vi "movement back by santimeters.vi"(8 "error in (no error)":errorcluster, 11 "range in santimeters":dbl format="%#_13g") -> (0 "error out":errorcluster)   [LabVIEW 2017]
uses:
  <vilib>/myRIO/Common/Instrument Driver Framework/myRIO v1.0/Encoder/typedefs/Encoder Signal Mode.ctl
  <vilib>/myRIO/Instrument Drivers/Onboard IO/Encoder/typedefs/Encoder Reference.ctl
  <vilib>/myRIO/Common/Instrument Driver Framework/Utilities/typedefs/myRIO Generic Hardware Reference.ctl
  <vilib>/myRIO/Common/Instrument Driver Framework/Utilities/typedefs/Hardware Version Enum.ctl
  <vilib>/myRIO/Common/Instrument Driver Framework/Utilities/typedefs/myRIO v1.0 Reference.ctl
  <vilib>/myRIO/Common/Instrument Driver Framework/Utilities/typedefs/Generic FPGA Reference.ctl
  <vilib>/myRIO/Common/Instrument Driver Framework/myRIO v1.0/Encoder/typedefs/Encoder Channels Enum.ctl
  <vilib>/myRIO/Common/Instrument Driver Framework/myRIO v1.0/Encoder/typedefs/Encoder Configuration v1.0.ctl
  <vilib>/userdefined/High Color/nirio_resource_hc.ctl
  <vilib>/myRIO/Instrument Drivers/Onboard IO/I2C/typedefs/I2C Reference.ctl
  <vilib>/myRIO/Common/Instrument Driver Framework/myRIO v1.0/I2C/typedefs/I2C Channels Enum.ctl
  <vilib>/myRIO/Instrument Drivers/Onboard IO/I2C/typedefs/I2C Configuration.ctl
  <vilib>/myRIO/Instrument Drivers/Onboard IO/I2C/typedefs/I2C Transfer Rate.ctl
  <vilib>/myRIO/Common/Instrument Driver Framework/Utilities/vis/Is FPGA Ref Available.vi
  <vilib>/myRIO/Common/Instrument Driver Framework/myRIO v1.0/Encoder/vis/myRIO v1.1 Open Encoder.vi
  <vilib>/myRIO/Instrument Drivers/Onboard IO/Encoder/vis/Read.vi
  <vilib>/myRIO/Common/Instrument Driver Framework/myRIO v1.0/I2C/vis/myRIO v1.1 Open I2C.vi
  <vilib>/myRIO/Common/Instrument Driver Framework/Utilities/vis/Validate Channels.vi
  <vilib>/myRIO/Common/Instrument Driver Framework/myRIO v1.0/Encoder/vis/myRIO v1.0 Reserve Encoder.vi
  <vilib>/myRIO/Common/Instrument Driver Framework/myRIO v1.0/I2C/vis/myRIO v1.0 Reserve I2C.vi
  <vilib>/myRIO/Common/Instrument Driver Framework/myRIO v1.0/I2C/vis/myRIO v1.0 Close I2C.vi
  <vilib>/myRIO/Common/Instrument Driver Framework/myRIO v1.0/Encoder/vis/myRIO v1.0 Build MUX Configuration Encoder.vi
  <vilib>/myRIO/Common/Instrument Driver Framework/myRIO v1.0/Resource Manager/vis/myRIO v1.0 Reserve Channel List.vi
  <vilib>/myRIO/Common/Instrument Driver Framework/myRIO v1.0/I2C/vis/myRIO v1.0 Build MUX Configuration I2C.vi
  <vilib>/myRIO/Common/Instrument Driver Framework/myRIO v1.0/I2C/vis/myRIO v1.0 Unreserve I2C.vi
  <vilib>/myRIO/Common/Instrument Driver Framework/myRIO v1.0/Resource Manager/vis/myRIO v1.0 Create Configuration List.vi
  <vilib>/myRIO/Common/Instrument Driver Framework/myRIO v1.0/Resource Manager/vis/myRIO v1.0 Reserve Channel.vi
  <vilib>/myRIO/Common/Instrument Driver Framework/myRIO v1.0/Resource Manager/vis/myRIO v1.0 Unreserve Channel.vi
  <vilib>/myRIO/Common/Instrument Driver Framework/myRIO v1.0/Resource Manager/vis/myRIO v1.0 Unreserve Channel List.vi
  <vilib>/myRIO/Common/Instrument Driver Framework/myRIO v1.0/Resource Manager/vis/myRIO v1.0 Build Mutex Name.vi
  <vilib>/Utility/VariantDataType/GetNumericInfo.vi
  <vilib>/Utility/error.llb/Error Cluster From Error Code.vi
  <vilib>/myRIO/Common/Instrument Driver Framework/myRIO v1.0/myRIO v1.1 Open.vi
  <vilib>/myRIO/Common/Instrument Driver Framework/Utilities/vis/IO Manager.vi
  <vilib>/myRIO/Common/Instrument Driver Framework/Utilities/vis/Configuration Manager.vi
  <vilib>/myRIO/Common/Instrument Driver Framework/myRIO v1.0/Resource Manager/vis/myRIO v1.0 Configure IO.vi
  <vilib>/myRIO/Common/Instrument Driver Framework/myRIO v1.0/myRIO v1.0 Close.vi
  <vilib>/myRIO/Common/Instrument Driver Framework/myRIO v1.0/Encoder/vis/myRIO v1.0 Configure Encoder.vi
  <vilib>/myRIO/Common/Instrument Driver Framework/myRIO v1.0/Encoder/vis/myRIO v1.0 Read Encoder.vi
  <vilib>/myRIO/Common/Instrument Driver Framework/myRIO v1.0/DIO/vis/myRIO v1.0 Write DIO.vi
  <vilib>/myRIO/Common/Instrument Driver Framework/myRIO v1.0/I2C/vis/myRIO v1.0 Shutdown I2C.vi
  <vilib>/myRIO/Instrument Drivers/Onboard IO/I2C/vis/myRIO I2C Open.xnode
  <vilib>/myRIO/Express VI/Onboard IO/Encoder/Encoder Express VI.xnode
  <vilib>/myRIO/Instrument Drivers/Onboard IO/Encoder/vis/myRIO Encoder Open.xnode
  <vilib>/myRIO/Instrument Drivers/Onboard IO/I2C/I2C.lvlib
  <vilib>/myRIO/Instrument Drivers/Onboard IO/Encoder/Encoder.lvlib
  <vilib>/myRIO/Instrument Drivers/Onboard IO/DIO/DIO.lvlib
panel:
  out "main angle":ext
  out "axis Z(after)":ext
  out "zero angle":ext
  out "left":dbl
  out "right":dbl
  out "axis Z(paste)":ext
  in  "Stop Button":bool
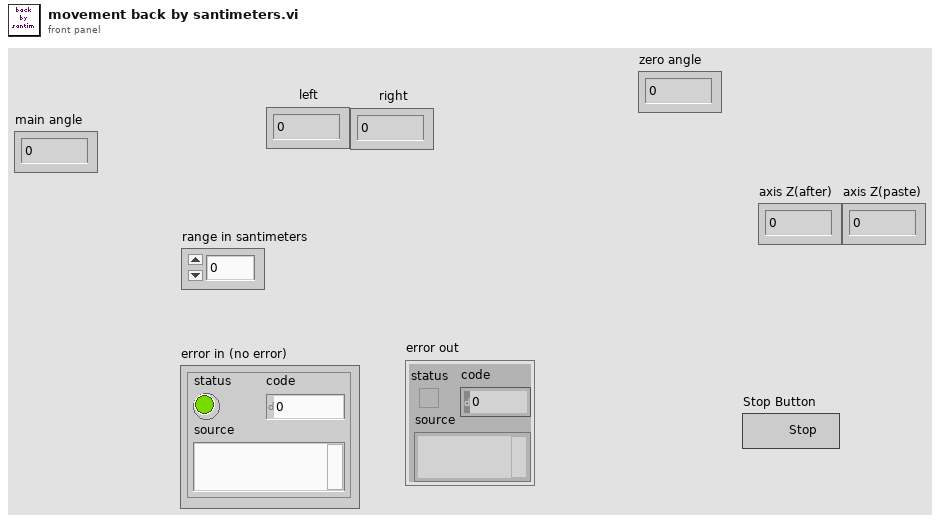
[diagram p1: front panel]
types:
  T1 = typedef "DIO.lvlib/DIO Reference.ctl" = cluster{"myRIO Reference":T2, "DIO Channels List":T6}
  T2 = typedef "myRIO Generic Hardware Reference.ctl" = cluster{"myRIO Model":T3, "myRIO Hardware Reference":T4}
  T3 = typedef "Hardware Version Enum.ctl" = enum16{"Unknown", "myRIO-1900", "myRIO-1950", "roboRIO", "NI ELVIS RIO CM"}
  T4 = typedef "myRIO v1.0 Reference.ctl" = cluster{"Generic FPGA Reference":T5, "Allow multiple opens":bool}
  T5 = typedef "Generic FPGA Reference.ctl" = refnum<k20>
  T6 = typedef "DIO Channels List.ctl" = T7[]
  T7 = typedef "DIO Channels Enum.ctl" = enum16{"Not Connected", "C/DIO0", "C/DIO1", "C/DIO2", "C/DIO3", "C/DIO4", "C/DIO5", "C/DIO6", "C/DIO7", "A/DIO0", "A/DIO1", "A/DIO2", "A/DIO3", "A/DIO4", "A/DIO5", "A/DIO6", "A/DIO7", "A/DIO8", "A/DIO9", "A/DIO10", "A/DIO11", "A/DIO12", "A/DIO13", "A/DIO14", "A/DIO15", "B/DIO0", "B/DIO1", "B/DIO2", "B/DIO3", "B/DIO4", "B/DIO5", "B/DIO6", "B/DIO7", "B/DIO8", "B/DIO9", "B/DIO10", "B/DIO11", "B/DIO12", "B/DIO13", "B/DIO14", "B/DIO15", "LED0", "LED1", "LED2", "LED3", "Button0", "DIO/DIO0", "DIO/DIO1", "DIO/DIO2", "DIO/DIO3", "DIO/DIO4", "DIO/DIO5", "DIO/DIO6", "DIO/DIO7", "DIO/DIO8", "DIO/DIO9", "SPI/CS0", "SPI/CS1", "SPI/CS2", "SPI/CS3", "LED RADIO (Green)", "LED RADIO (Red)", "LED COMM (Green)", "LED COMM (Red)", "LED MODE (Green)", "LED MODE (Red)"}
  T8 = typedef "I2C.lvlib/I2C Reference.ctl" = cluster{"myRIO Reference":T2, "I2C Channels Enum":T9, "I2C Configuration":T10}
  T9 = typedef "I2C Channels Enum.ctl" = enum16{"Not Connected", "A/I2C", "B/I2C", "I2C/I2C"}
  T10 = typedef "I2C.lvlib/I2C Configuration.ctl" = cluster{"I2C Transfer Rate":T11}
  T11 = typedef "I2C.lvlib/I2C Transfer Rate.ctl" = enum16{"Standard mode (100 kbps)", "Fast mode (400 kbps)"}
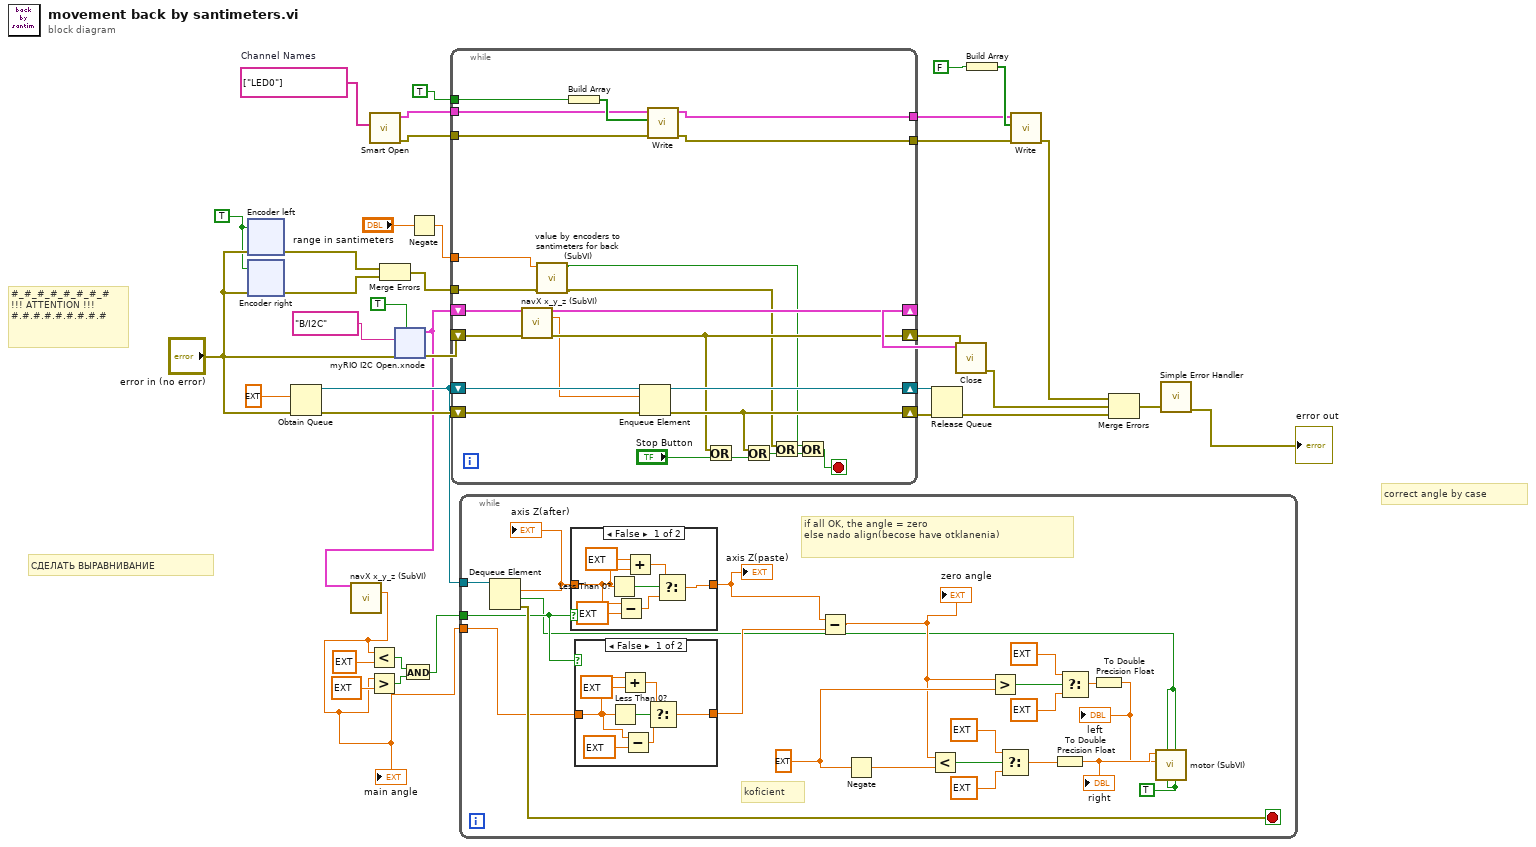
[diagram p0: block diagram]
diagram:
  w9 = tag[] ["LED0"]  # Channel Names
  w10 = TRUE ("Reset Counter")
  # "СДЕЛАТЬ ВЫРАВНИВАНИЕ"
  # "correct angle by case"
  # "#_#_#_#_#_#_#_#\n!!! ATTENTION !!!\n#.#.#.#.#.#.#.#.#"
  n1 = xnode ("Encoder left")("error in (no error)"="error in (no error)", "Reset Counter"=w10) -> ("error out"=w15:errorcluster)  [unwired: 3 out]
  n2 = xnode ("Encoder right")("error in (no error)"="error in (no error)", "Reset Counter"=w10) -> ("error out"=w14:errorcluster)  [unwired: 3 out]
  n3 = Obtain Queue(element data type=ext 0.0 ("value Z"), error in (no error)="error in (no error)") -> (queue out=w25:refnum<queue>, error out=w37:errorcluster)  [unwired: 3 in, 1 out]
  n4 = call <vilib>:"Smart Open.vi"("Channel Names"=w9) -> ("error out"=w4:errorcluster, "DIO Ref Out"=w5:T1)  [unwired: 9 in]
  n5 = Merge Errors(w15, w14) -> (w13:errorcluster)
  n6 = xnode "myRIO I2C Open.xnode"("error in (no error)"="error in (no error)", "Allow multiple opens?"=TRUE, "Channel Name"=tag "B/I2C") -> ("error out"=w30:errorcluster, "I2C Ref Out"=w23:T8)
  n7 = call "navX x_y_z (SubVI).vi"("I2C Ref Out in"=w23) -> ("value Z"=w20:ext)  [unwired: 10 in, 4 out]
  "main angle" <- w20
  n8 = Less?(x=w20, y=ext 90.0) -> (x < y?=w18:bool)
  n9 = Greater?(x=w20, y=ext -90.0) -> (0:w21:bool)
  n10 = And(x=w18, y=w21) -> (x .and. y?=w17:bool)
  n11 = Negate(x="range in santimeters") -> (-x=w11:dbl)
  n12 = while {
    shift-right: [w55] -> w35
    shift-left: w37 -> [w60]
    shift-right: [w59] -> w36
    shift-left: w25 -> [w61]
    shift-right: [w56] -> w31
    shift-left: w23 -> [w57]
    shift-right: [w52] -> w29
    shift-left: w30 -> [w53]
    tunnel: w13 -> [w44]
    tunnel: w11 -> [w47]
    tunnel: TRUE -> [w43]
    tunnel: w5 -> [w41]
    tunnel: w4 -> [w40]
    tunnel: [w39] -> w3
    tunnel: [w38] -> w2
    stop <- w49 stop-if-true
    n13 = call "navX x_y_z (SubVI).vi"("I2C Ref Out in"=w57, "error in (no error)"=w53) -> ("I2C Ref Out out"=w56:T8, "value Z"=w51:ext, "error out"=w52:errorcluster)  [unwired: 9 in, 2 out]
    n14 = call "value by encoders to santimeters for back (SubVI).vi"("error in (no error)"=w44, "range in"=w47) -> ("error out"=w45:errorcluster, "value >= range"=w46:bool)  [unwired: 7 in, 1 out]
    n15 = Build Array(w43) -> (w42:bool[])
    n16 = Enqueue Element(queue=w61, element=w51, error in (no error)=w60) -> (queue out=w59:refnum<queue>, error out=w55:errorcluster)  [unwired: 1 in, 1 out]
    n17 = call <vilib>:"Write.vi"("error in (no error)"=w40, "Values"=w42, "DIO Ref In"=w41) -> ("error out"=w38:errorcluster, "DIO Ref Out"=w39:T1)  [unwired: 6 in]
    n18 = Or(x=w52, y="Stop Button") -> (x .or. y?=w54:bool)
    n19 = Or(x=w55, y=w54) -> (x .or. y?=w50:bool)
    n20 = Or(x=w45, y=w50) -> (x .or. y?=w48:bool)
    n21 = Or(x=w46, y=w48) -> (x .or. y?=w49:bool)
  }
  n22 = while {
    tunnel: w25 -> [w83]
    tunnel: w20 -> [w67]
    tunnel: w17 -> [w66]
    stop <- w82 stop-if-true
    w65 = TRUE ("M1 (Pin 26)")
    w75 = ext 1.0 ("y")
    # "koficient"
    # "if all OK, the angle = zero\nelse nado align(becose have otklanenia)"
    n23 = Dequeue Element(queue=w83) -> (element=w69:ext, timed out?=w64:bool, error out=w82:errorcluster)  [unwired: 2 in, 1 out]
    "axis Z(after)" <- w69
    n24 = case shown="False" w66 {
      tunnel: [w97 w99] -> w70
      tunnel: w69 -> [w93 w99]
      frame False {
        n25 = Less Than 0?(x=w93) -> (x < 0?=w98:bool)
        n26 = Subtract(x=w93, y=ext 180.0) -> (x-y=w94:ext)
        n27 = Add(x=ext 180.0, y=w93) -> (x+y=w96:ext)
        n28 = Select(t=w96, s=w98, f=w94) -> (s? t:f=w97:ext)
      }
      frame True {
      }
    }
    "axis Z(paste)" <- w70
    n29 = case shown="False" w66 {
      tunnel: [w89 w91] -> w68
      tunnel: w67 -> [w86 w91]
      frame False {
        n30 = Less Than 0?(x=w86) -> (x < 0?=w90:bool)
        n31 = Add(x=w86, y=ext 180.0) -> (x+y=w88:ext)
        n32 = Subtract(x=w86, y=ext 180.0) -> (x-y=w87:ext)
        n33 = Select(t=w88, s=w90, f=w87) -> (s? t:f=w89:ext)
      }
      frame True {
      }
    }
    n34 = Subtract(x=w70, y=w68) -> (x-y=w71:ext)
    "zero angle" <- w71
    n35 = Negate(x=w75) -> (-x=w74:ext)
    n36 = Less?(x=w71, y=w74) -> (x < y?=w78:bool)
    n37 = Greater?(x=w71, y=w75) -> (0:w81:bool)
    n38 = Select(t=ext 0.2 ("y"), s=w78, f=ext 0.30000000000000000001 ("y")) -> (s? t:f=w72:ext)
    n39 = To Double Precision Float(number=w72) -> (double precision float=w63:dbl)
    "right" <- w63
    n40 = Select(t=ext 0.2 ("y"), s=w81, f=ext 0.30000000000000000001 ("y")) -> (s? t:f=w73:ext)
    n41 = To Double Precision Float(number=w73) -> (double precision float=w62:dbl)
    "left" <- w62
    n42 = call "motor (SubVI).vi"("M1 (Pin 26)"=w65, "M1 (Pin 25)"=w64, "M0 (Pin 23)"=w65, "M0 (Pin 21)"=w64, "PWM1"=w62, "PWM0"=w63) -> ()  [unwired: 5 in, 1 out]
  }
  n43 = Release Queue(queue=w36, error in (no error)=w35) -> (error out=w26:errorcluster)  [unwired: 1 in, 2 out]
  n44 = call <vilib>:"Close.vi"("error in (no error)"=w29, "I2C Ref In"=w31) -> ("error out"=w27:errorcluster)  [unwired: 9 in]
  n45 = Build Array(FALSE) -> (w8:bool[])
  n46 = call <vilib>:"Write.vi"("error in (no error)"=w2, "Values"=w8, "DIO Ref In"=w3) -> ("error out"=w1:errorcluster)  [unwired: 6 in, 1 out]
  n47 = Merge Errors(w1, w27, w26) -> (w28:errorcluster)
  n48 = call <vilib>:"Simple Error Handler.vi"("error in (no error)"=w28) -> ("error out"=→"error out":errorcluster)  [unwired: 4 in, 4 out]
